vi "GetState_TestStand.vi"(6 "error in (no error)":errorcluster, 7 "Calibrate?":bool, 8 "IMU Channel":tag="A/I2C") -> (0 "error out":errorcluster, 2 "Angular Velocity":dbl[](array[numeric]), 3 "imu accel":i16[](array[numeric]))   [LabVIEW 2019]
uses:
  <vilib>/Analysis/baseanly.llb/Mean (DBL).vi
  <vilib>/Analysis/NI_AALBase.lvlib
panel:
  out "error out 2":errorcluster
  out "Acceleration":dbl[](array[numeric])
  in  "Acceleration Factor (experimentally determined)":dbl format="%#_13g"
  out "MyRIO Acceleration":dbl[](array[numeric])
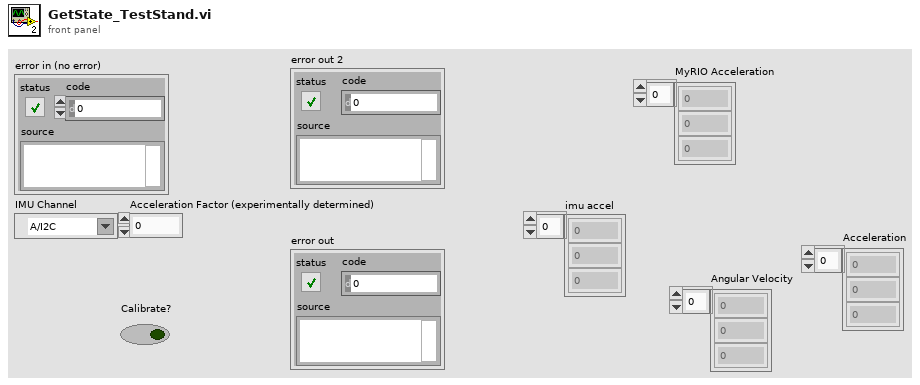
[diagram p1: front panel]
types:
  T1 = cluster{"X-axis":i16, "Y-axis":i16, "Z-axis":i16}
  T2 = cluster{"X-Axis":dbl, "Y-Axis":dbl, "Z-Axis":dbl}
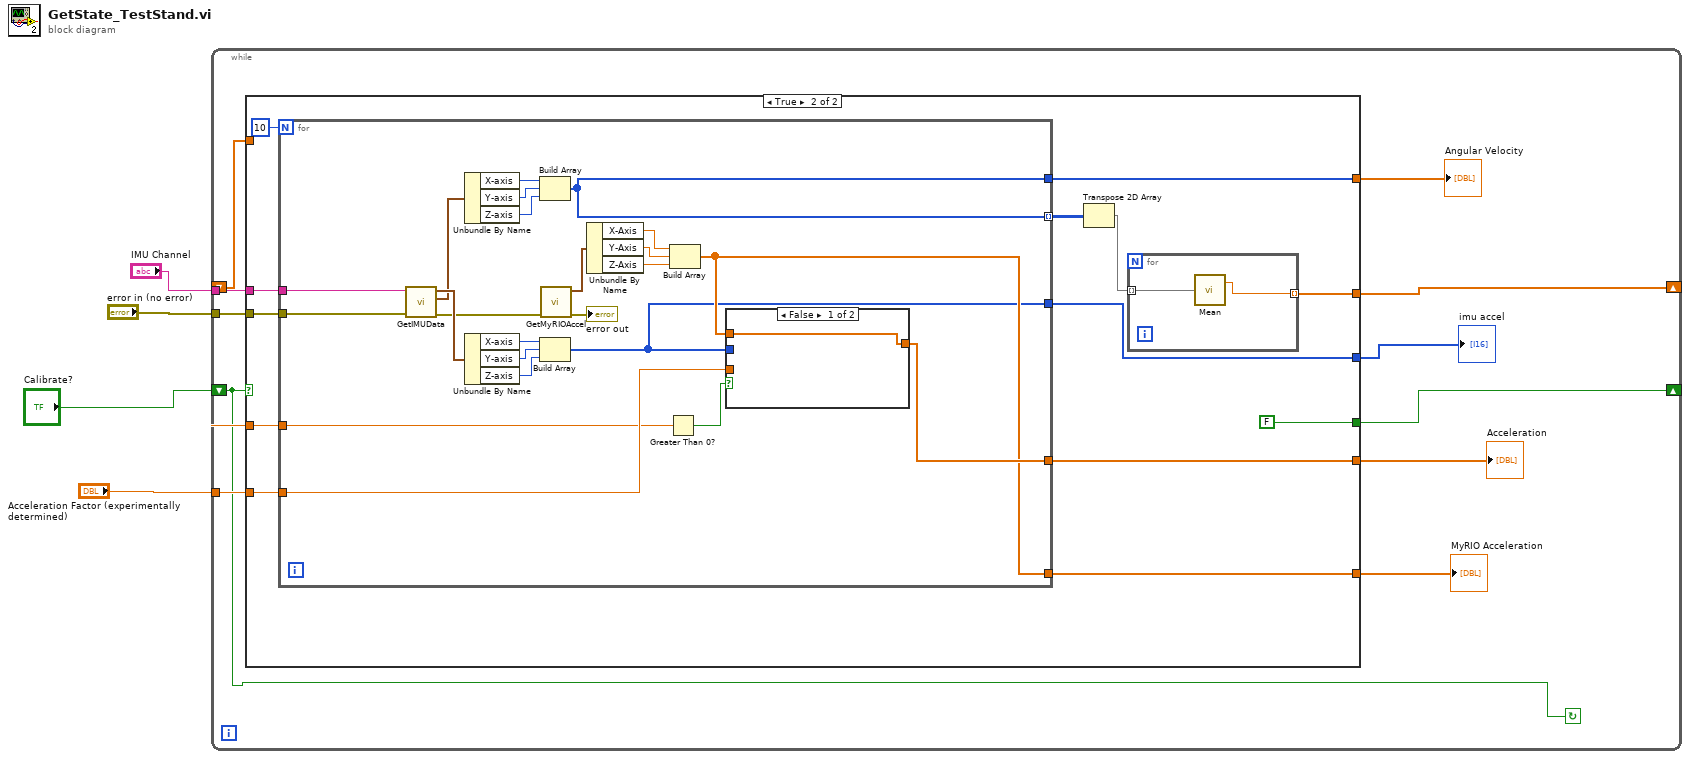
[diagram p0: block diagram]
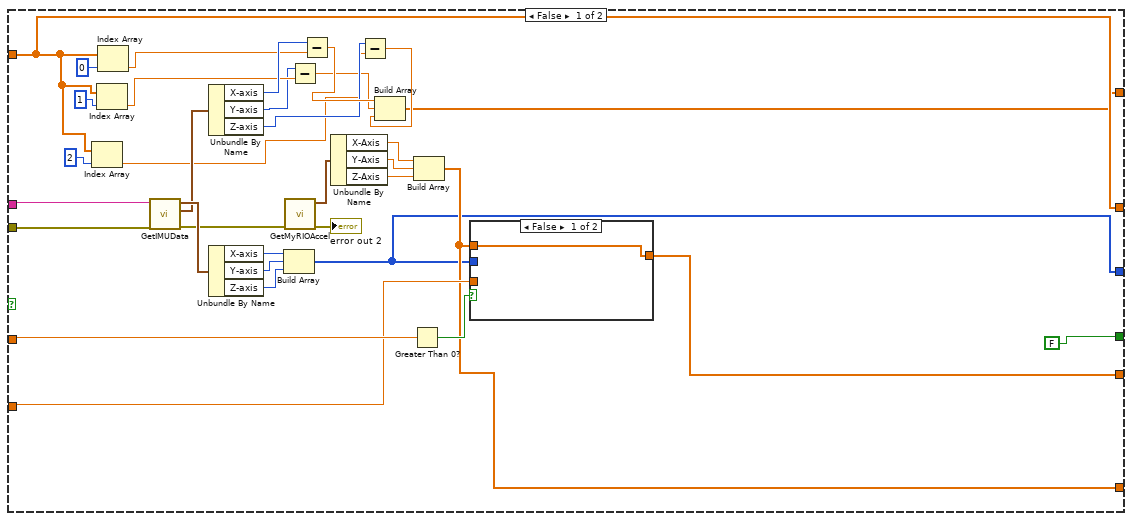
[diagram p2: hidden frame]
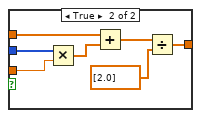
[diagram p3: hidden frame]
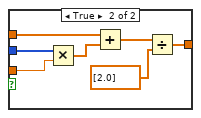
[diagram p4: hidden frame]
diagram:
  n1 = while {
    tunnel: "error in (no error)" -> [w15]
    tunnel: "IMU Channel" -> [w14]
    tunnel: "Acceleration Factor (experimentally determined)" -> [w13]
    shift-right: [w12] -> _
    shift-left: "Calibrate?" -> [w5]
    shift-right: [w11] -> _
    shift-left: _ -> [w10]
    stop <- w5 continue-if-true
    n2 = case shown="True" w5 {
      tunnel: w15 -> [w37 w70]
      tunnel: w14 -> [w38 w69]
      tunnel: w13 -> [w35 w68]
      tunnel: w13 -> [w36 w67]
      tunnel: [FALSE FALSE] -> w12
      tunnel: [w22 w62] -> w11
      tunnel: w10 -> [w22 _]
      tunnel: [w17 w61] -> w9
      tunnel: [w20 w60] -> w8
      tunnel: [w19 w59] -> w7
      tunnel: [w18 w58] -> w6
      frame False {
        n3 = Index Array(array=w22, index=2) -> (element=w25:dbl)
        n4 = Index Array(array=w22, index=1) -> (element=w28:dbl)
        n5 = Index Array(array=w22, index=0) -> (element=w32:dbl)
        n6 = call "GetIMUData.vi"("error in (no error)"=w37, "Channel Name"=w38) -> ("error out"=w16:errorcluster, "GyroData"=w46:T1, "AccelData"=w47:T1)  [unwired: 7 in]
        n7 = Unbundle By Name(w46) -> ("X-axis"=w33:i16, "Y-axis"=w27:i16, "Z-axis"=w26:i16)
        n8 = Unbundle By Name(w47) -> ("X-axis"=w42:i16, "Y-axis"=w41:i16, "Z-axis"=w40:i16)
        n9 = Build Array(w42, w41, w40) -> (w18:i16[])
        n10 = call "GetMyRIOAccel.vi"("error in (no error)"=w16) -> ("error out"=→"error out 2":errorcluster, "output cluster"=w48:T2)  [unwired: 9 in]
        n11 = Subtract(x=w27, y=w28) -> (x-y=w24:dbl)
        n12 = Subtract(x=w33, y=w32) -> (x-y=w31:dbl)
        n13 = Unbundle By Name(w48) -> ("X-Axis"=w45:dbl, "Y-Axis"=w44:dbl, "Z-Axis"=w43:dbl)
        n14 = Subtract(x=w26, y=w25) -> (x-y=w23:dbl)
        n15 = Build Array(w31, w24, w23) -> (w17:dbl[])
        n16 = Greater Than 0?(x=w36) -> (x > 0?=w39:bool)
        n17 = Build Array(w45, w44, w43) -> (w19:dbl[])
        n18 = case shown="False" w39 {
          tunnel: w35 -> [_ w57]
          tunnel: w18 -> [_ w56]
          tunnel: w19 -> [w50 w54]
          tunnel: [w50 w51] -> w20
          frame False {
          }
          frame True {
            n19 = Multiply(x=w56, y=w57) -> (x*y=w55:dbl[])
            n20 = Add(x=w54, y=w55) -> (x+y=w53:dbl[])
            n21 = Divide(x=w53, y=dbl[] [2.0]) -> (x/y=w51:dbl[])
          }
        }
      }
      frame True {
        n22 = for {
          N: 10 -> [_]
          tunnel: [w77] -> w65 mode=indexing
          tunnel: w70 -> [w81]
          tunnel: w69 -> [w80]
          tunnel: w68 -> [w79]
          tunnel: w67 -> [w78]
          tunnel: [w77] -> w61
          tunnel: [w76] -> w60
          tunnel: [w75] -> w59
          tunnel: [w74] -> w58
          n23 = call "GetIMUData.vi"("error in (no error)"=w81, "Channel Name"=w80) -> ("error out"=w73:errorcluster, "GyroData"=w92:T1, "AccelData"=w93:T1)  [unwired: 7 in]
          n24 = Unbundle By Name(w92) -> ("X-axis"=w88:i16, "Y-axis"=w87:i16, "Z-axis"=w86:i16)
          n25 = Unbundle By Name(w93) -> ("X-axis"=w85:i16, "Y-axis"=w84:i16, "Z-axis"=w83:i16)
          n26 = Build Array(w88, w87, w86) -> (w77:i16[])
          n27 = Build Array(w85, w84, w83) -> (w74:i16[])
          n28 = call "GetMyRIOAccel.vi"("error in (no error)"=w73) -> ("error out"=→"error out":errorcluster, "output cluster"=w94:T2)  [unwired: 9 in]
          n29 = Unbundle By Name(w94) -> ("X-Axis"=w91:dbl, "Y-Axis"=w90:dbl, "Z-Axis"=w89:dbl)
          n30 = Greater Than 0?(x=w78) -> (x > 0?=w82:bool)
          n31 = Build Array(w91, w90, w89) -> (w75:dbl[])
          n32 = case shown="False" w82 {
            tunnel: w79 -> [_ w103]
            tunnel: w74 -> [_ w102]
            tunnel: w75 -> [w96 w100]
            tunnel: [w96 w97] -> w76
            frame False {
            }
            frame True {
              n33 = Multiply(x=w102, y=w103) -> (x*y=w101:dbl[])
              n34 = Add(x=w100, y=w101) -> (x+y=w99:dbl[])
              n35 = Divide(x=w99, y=dbl[] [2.0]) -> (x/y=w97:dbl[])
            }
          }
        }
        n36 = Transpose 2D Array(2D array=w65) -> (transposed array=w64:i16[][])
        n37 = for {
          tunnel: w64 -> [w72] mode=indexing
          tunnel: [w71] -> w62 mode=indexing
          n38 = call-poly <vilib>:"Mean.vi"("X"=w72) -> ("mean"=w71:dbl)  [unwired: 1 out]
        }
      }
    }
    "Angular Velocity" <- w9
    "Acceleration" <- w8
    "MyRIO Acceleration" <- w7
    "imu accel" <- w6
  }
